vi "Get All Clients.vi"(8 "error in (no error)":errorcluster, 11 "TCP Server in":refnum<class "TCP Server.lvclass">) -> (0 "error out":errorcluster, 2 "Clients":refnum<class "TCP Client.lvclass">[](array[class]), 3 "TCP Server out":refnum<class "TCP Server.lvclass">)   [LabVIEW 2012, in "Stream-TCP.lvlib" / "TCP Server.lvclass"]
uses:
  TCP Server.lvclass
  TCP Client/TCP Client.lvclass
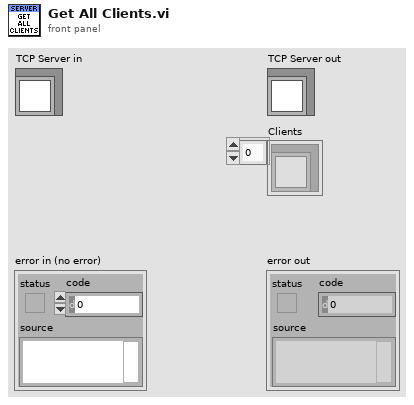
[diagram p1: front panel]
types:
  T1 = typedef "Stream-TCP.lvlib/TCP Server.lvclass/Ref Data.ctl" = cluster{"Listener":refnum<k5>, "Clients":refnum<class "TCP Client.lvclass">[], "Server Loop":bool}
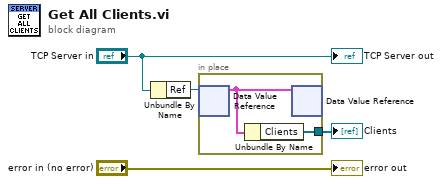
[diagram p0: block diagram]
diagram:
  n1 = Unbundle By Name("TCP Server in") -> ("Ref"=w3:refnum<data-value>)
  n2 = in-place {
    in-place-border: [w5] -> w1
    n3 = in-place-dvr #1(w3) -> (w6:T1)  [unwired: 1 out]
    n4 = Unbundle By Name(w6) -> ("Clients"=w5:refnum<class "TCP Client.lvclass">[])
    n5 = in-place-dvr #1(w6) -> ()  [unwired: 2 out]
  }
  "Clients" <- w1
  "error out" <- "error in (no error)"
  "TCP Server out" <- "TCP Server in"
